vi "Display.vi"(0 "STEP in":refnum<class "STEP.lvclass">, 2 "Alarms triggered?":T3, 3 "STEP State":T4, 4 "Current Sequence":T1, 5 "error in (no error)":errorcluster, 9 "SEQ STEP Display":refnum<notifier>) -> (14 "STEP out":refnum<class "STEP.lvclass">, 19 "error out":errorcluster)   [LabVIEW 2014, in "SeqLoop.lvlib" / "STEP Classes.lvlib" / "STEP.lvclass"]
doc: "Gestiona el envío de Datos al Display."
uses:
  STEP.lvclass
  TypeDefs/STEP State.ctl
  TypeDefs/STEP Display.ctl
  Mimico Display/TypeDefs/Mimic Data.ctl
  Mimico Display/TypeDefs/BG Image.ctl
  Mimico Display/TypeDefs/mObject.ctl
  TypeDefs/Sequence.ctl
  TypeDefs/LogicParsedExpression.ctl
  STEP.lvclass/STEP.ctl
  Mimico Display/Mimico Display.lvlib
  SeqLoop.lvlib
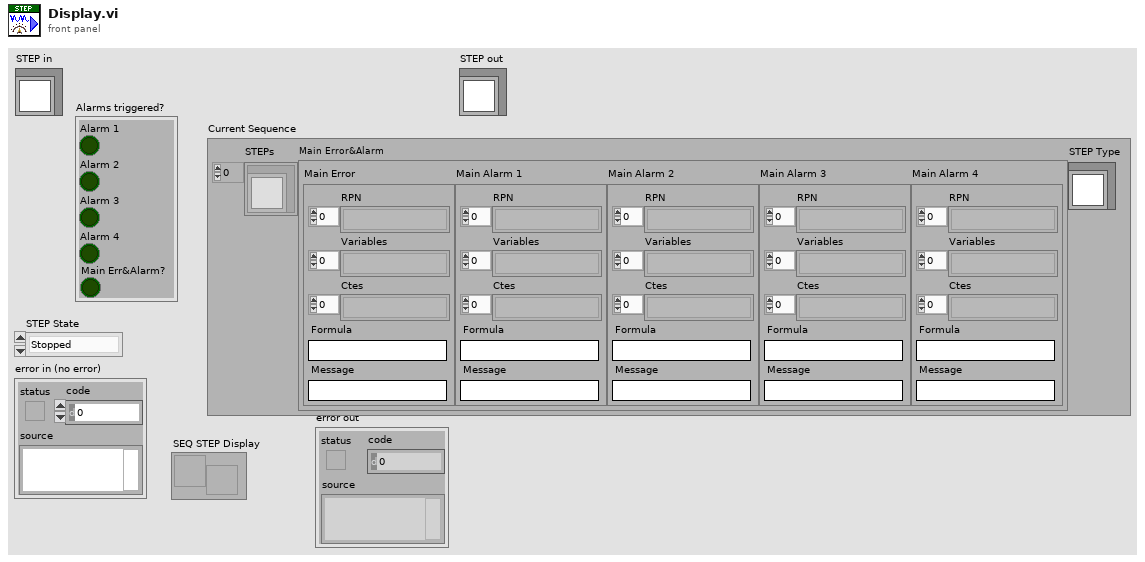
[diagram p1: front panel]
types:
  T1 = typedef "SeqLoop.lvlib/Sequence.ctl" = cluster{"STEPs":refnum<class "STEP.lvclass">[], "Main Error&Alarm":cluster{"Main Error":T2, "Main Alarm 1":T2, "Main Alarm 2":T2, "Main Alarm 3":T2, "Main Alarm 4":T2}, "STEP Type":refnum<class "STEP.lvclass">}
  T2 = typedef "SeqLoop.lvlib/LogicParsedExpression.ctl" = cluster{"RPN ":string[], "Variables":string[], "Ctes":string[], "Formula":string, "Message":string}
  T3 = cluster{"Alarm 1":bool, "Alarm 2":bool, "Alarm 3":bool, "Alarm 4":bool, "Main Err&Alarm?":bool}
  T4 = typedef "SeqLoop.lvlib/STEP State.ctl" = enum16{"Stopped", "First Call", "Idle...", "Advance OK", "Alarm", "Output Security", "Error"}
  T5 = typedef "STEP Display.ctl" = cluster{"Mimic Data":T6, "Operator Mssg":string, "Error":cluster{"true?":bool, "Message":string}, "Alarm 1":cluster{"true?":bool, "Message":string}, "Alarm 2":cluster{"true?":bool, "Message":string}, "Alarm 3":cluster{"true?":bool, "Message":string}, "Alarm 4":cluster{"true?":bool, "Message":string}}
  T6 = typedef "SeqLoop.lvlib/Mimico Display.lvlib/Mimic Data.ctl" = cluster{"BG Image":T7, "Mimic mObjects":T8[]}
  T7 = typedef "SeqLoop.lvlib/Mimico Display.lvlib/BG Image.ctl" = cluster{"Path":path, "point":cluster{"x":i16, "y":i16}}
  T8 = typedef "SeqLoop.lvlib/Mimico Display.lvlib/mObject.ctl" = cluster{"point":cluster{"x":i16, "y":i16}, "Precision (Digits)":i32, "Visible?":bool, "Ref":string, "Comment":string}
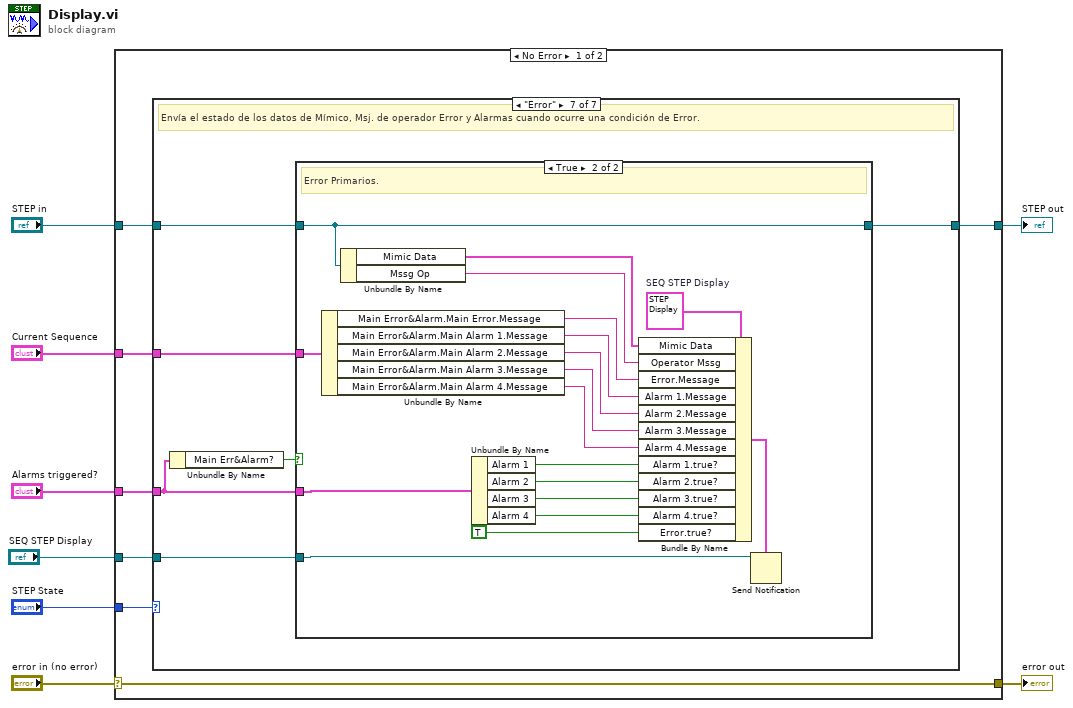
[diagram p0: block diagram]
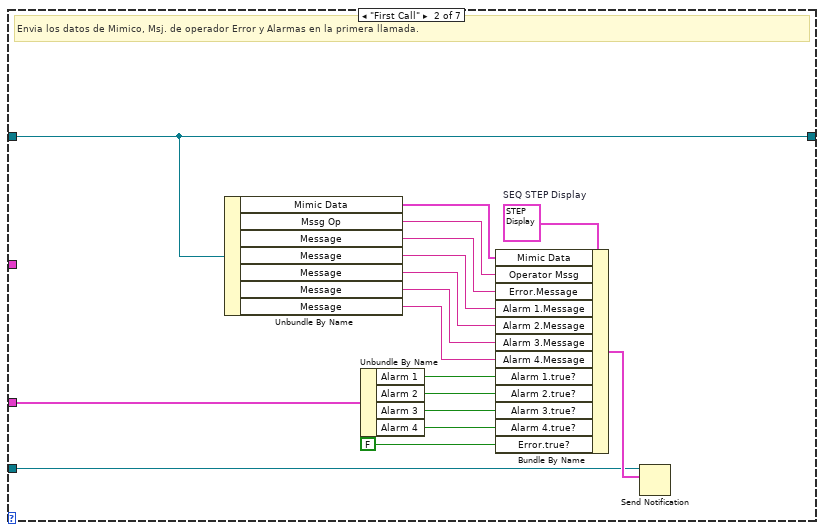
[diagram p3: hidden frame]
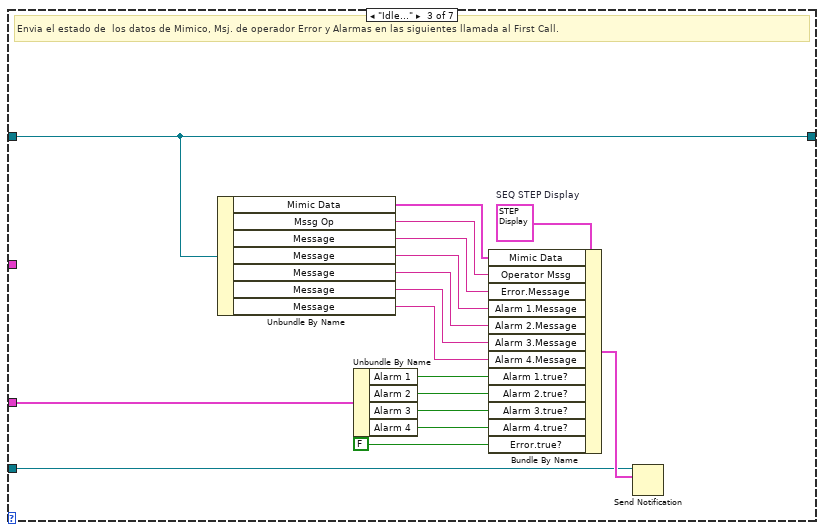
[diagram p4: hidden frame]
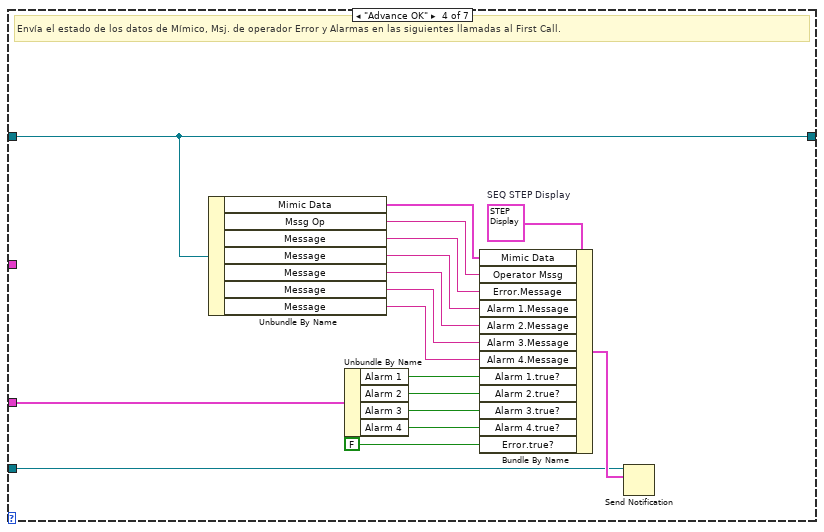
[diagram p5: hidden frame]
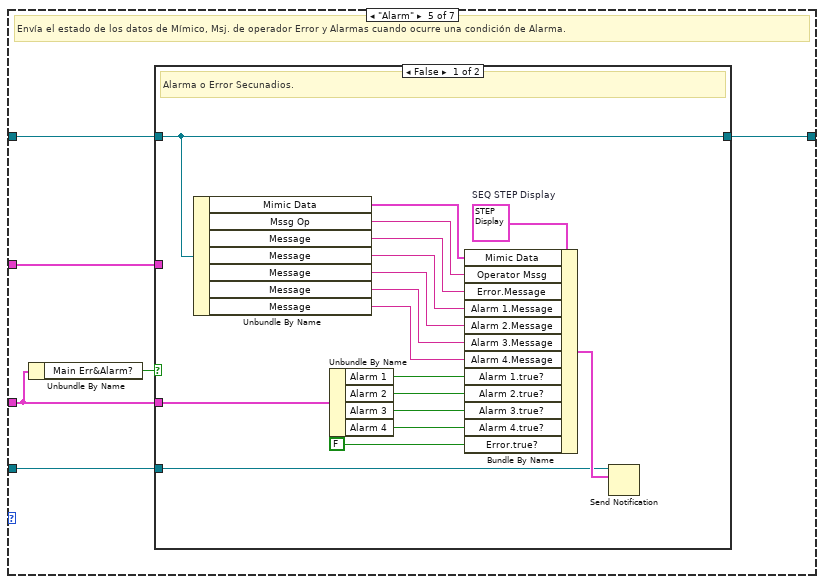
[diagram p6: hidden frame]
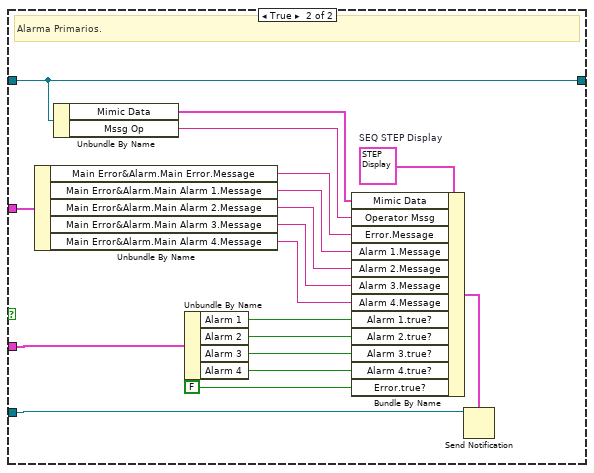
[diagram p7: hidden frame]
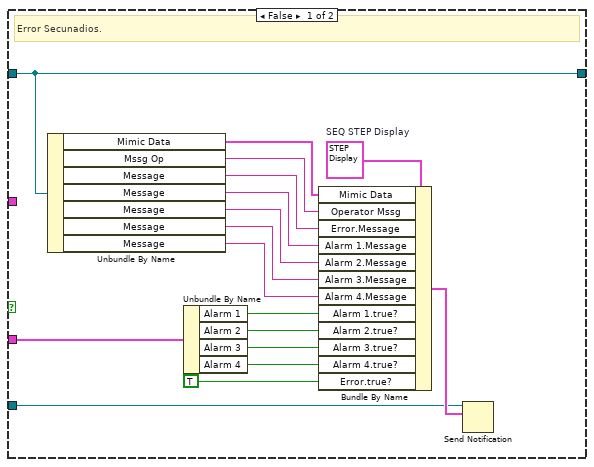
[diagram p9: hidden frame]
diagram:
  n1 = case shown="No Error" "error in (no error)" {
    selector: "error in (no error)" -> [w15 w152]
    tunnel: [w15 w152] -> w7
    tunnel: [w13 w151] -> w5
    tunnel: "STEP in" -> [w14 w151]
    tunnel: "STEP State" -> [w12 _]
    tunnel: "Alarms triggered?" -> [w11 _]
    tunnel: "SEQ STEP Display" -> [w10 _]
    tunnel: "Current Sequence" -> [w9 _]
    frame No Error {
      n2 = case shown="\"Error\"" w12 {
        tunnel: w14 -> [w16 w17 w34 w52 w72 w109 w115]
        tunnel: [w16 w17 w34 w52 w68 w109 w110] -> w13
        tunnel: w11 -> [_ w18 w36 w53 w70 _ w113]
        tunnel: w10 -> [_ w19 w35 w51 w69 _ w114]
        tunnel: w9 -> [_ _ _ _ w71 _ w111]
        frame "Stopped", Default {
        }
        frame "First Call" {
          w33 = T5 {"Mimic Data"={"BG Image"={"Path"=path "", "point"={"x"=0, "y"=0}}, "Mimic mObjects"=[]}, "Operator Mssg"="", "Error"={"true?"=FALSE, "Message"=""}, "Alarm 1"={"true?"=FALSE, "Message"=""}, "Alarm 2"={"true?"=FALSE, "Message"=""}, "Alarm 3"={"true?"=FALSE, "Message"=""}, "Alarm 4"={"true?"=FALSE, "Message"=""}}  # SEQ STEP Display
          # "Envia los datos de Mimico, Msj. de operador Error y Alarmas en la primera llamada."
          n3 = Unbundle By Name(w17) -> ("Mimic Data"=w32:T6, "Mssg Op"=w31:string, "Message"=w30:string, "Message"=w29:string, "Message"=w28:string, "Message"=w27:string, "Message"=w26:string)
          n4 = Unbundle By Name(w18) -> ("Alarm 1"=w25:bool, "Alarm 2"=w24:bool, "Alarm 3"=w23:bool, "Alarm 4"=w22:bool)
          n5 = Bundle By Name(cluster=w33, "Mimic Data"=w32, "Operator Mssg"=w31, "Error.Message"=w30, "Alarm 1.Message"=w29, "Alarm 2.Message"=w28, "Alarm 3.Message"=w27, "Alarm 4.Message"=w26, "Alarm 1.true?"=w25, "Alarm 2.true?"=w24, "Alarm 3.true?"=w23, "Alarm 4.true?"=w22, "Error.true?"=FALSE) -> (w21:T5)
          n6 = Send Notification(notification=w21, notifier=w19) -> ()  [unwired: 1 in, 2 out]
        }
        frame "Idle..." {
          w37 = T5 {"Mimic Data"={"BG Image"={"Path"=path "", "point"={"x"=0, "y"=0}}, "Mimic mObjects"=[]}, "Operator Mssg"="", "Error"={"true?"=FALSE, "Message"=""}, "Alarm 1"={"true?"=FALSE, "Message"=""}, "Alarm 2"={"true?"=FALSE, "Message"=""}, "Alarm 3"={"true?"=FALSE, "Message"=""}, "Alarm 4"={"true?"=FALSE, "Message"=""}}  # SEQ STEP Display
          # "Envia el estado de  los datos de Mimico, Msj. de operador Error y Alarmas en las siguientes llamada al First Call."
          n7 = Unbundle By Name(w34) -> ("Mimic Data"=w38:T6, "Mssg Op"=w39:string, "Message"=w40:string, "Message"=w41:string, "Message"=w42:string, "Message"=w43:string, "Message"=w44:string)
          n8 = Unbundle By Name(w36) -> ("Alarm 1"=w45:bool, "Alarm 2"=w46:bool, "Alarm 3"=w47:bool, "Alarm 4"=w48:bool)
          n9 = Bundle By Name(cluster=w37, "Mimic Data"=w38, "Operator Mssg"=w39, "Error.Message"=w40, "Alarm 1.Message"=w41, "Alarm 2.Message"=w42, "Alarm 3.Message"=w43, "Alarm 4.Message"=w44, "Alarm 1.true?"=w45, "Alarm 2.true?"=w46, "Alarm 3.true?"=w47, "Alarm 4.true?"=w48, "Error.true?"=FALSE) -> (w49:T5)
          n10 = Send Notification(notification=w49, notifier=w35) -> ()  [unwired: 1 in, 2 out]
        }
        frame "Advance OK" {
          w67 = T5 {"Mimic Data"={"BG Image"={"Path"=path "", "point"={"x"=0, "y"=0}}, "Mimic mObjects"=[]}, "Operator Mssg"="", "Error"={"true?"=FALSE, "Message"=""}, "Alarm 1"={"true?"=FALSE, "Message"=""}, "Alarm 2"={"true?"=FALSE, "Message"=""}, "Alarm 3"={"true?"=FALSE, "Message"=""}, "Alarm 4"={"true?"=FALSE, "Message"=""}}  # SEQ STEP Display
          # "Envía el estado de los datos de Mímico, Msj. de operador Error y Alarmas en las siguientes llamadas al First Call."
          n11 = Unbundle By Name(w52) -> ("Mimic Data"=w66:T6, "Mssg Op"=w65:string, "Message"=w64:string, "Message"=w63:string, "Message"=w62:string, "Message"=w61:string, "Message"=w60:string)
          n12 = Unbundle By Name(w53) -> ("Alarm 1"=w59:bool, "Alarm 2"=w58:bool, "Alarm 3"=w57:bool, "Alarm 4"=w56:bool)
          n13 = Bundle By Name(cluster=w67, "Mimic Data"=w66, "Operator Mssg"=w65, "Error.Message"=w64, "Alarm 1.Message"=w63, "Alarm 2.Message"=w62, "Alarm 3.Message"=w61, "Alarm 4.Message"=w60, "Alarm 1.true?"=w59, "Alarm 2.true?"=w58, "Alarm 3.true?"=w57, "Alarm 4.true?"=w56, "Error.true?"=FALSE) -> (w55:T5)
          n14 = Send Notification(notification=w55, notifier=w51) -> ()  [unwired: 1 in, 2 out]
        }
        frame "Alarm" {
          # "Envía el estado de los datos de Mímico, Msj. de operador Error y Alarmas cuando ocurre una condición de Alarma."
          n15 = Unbundle By Name(w70) -> ("Main Err&Alarm?"=w73:bool)
          n16 = case shown="False" w73 {
            tunnel: w72 -> [w74 w91]
            tunnel: w69 -> [w77 w94]
            tunnel: w70 -> [w75 w95]
            tunnel: w71 -> [_ w96]
            tunnel: [w74 w91] -> w68
            frame False {
              w90 = T5 {"Mimic Data"={"BG Image"={"Path"=path "", "point"={"x"=0, "y"=0}}, "Mimic mObjects"=[]}, "Operator Mssg"="", "Error"={"true?"=FALSE, "Message"=""}, "Alarm 1"={"true?"=FALSE, "Message"=""}, "Alarm 2"={"true?"=FALSE, "Message"=""}, "Alarm 3"={"true?"=FALSE, "Message"=""}, "Alarm 4"={"true?"=FALSE, "Message"=""}}  # SEQ STEP Display
              # "Alarma o Error Secunadios."
              n17 = Unbundle By Name(w74) -> ("Mimic Data"=w89:T6, "Mssg Op"=w88:string, "Message"=w87:string, "Message"=w86:string, "Message"=w85:string, "Message"=w84:string, "Message"=w83:string)
              n18 = Unbundle By Name(w75) -> ("Alarm 1"=w82:bool, "Alarm 2"=w81:bool, "Alarm 3"=w80:bool, "Alarm 4"=w79:bool)
              n19 = Bundle By Name(cluster=w90, "Mimic Data"=w89, "Operator Mssg"=w88, "Error.Message"=w87, "Alarm 1.Message"=w86, "Alarm 2.Message"=w85, "Alarm 3.Message"=w84, "Alarm 4.Message"=w83, "Alarm 1.true?"=w82, "Alarm 2.true?"=w81, "Alarm 3.true?"=w80, "Alarm 4.true?"=w79, "Error.true?"=FALSE) -> (w78:T5)
              n20 = Send Notification(notification=w78, notifier=w77) -> ()  [unwired: 1 in, 2 out]
            }
            frame True {
              w108 = T5 {"Mimic Data"={"BG Image"={"Path"=path "", "point"={"x"=0, "y"=0}}, "Mimic mObjects"=[]}, "Operator Mssg"="", "Error"={"true?"=FALSE, "Message"=""}, "Alarm 1"={"true?"=FALSE, "Message"=""}, "Alarm 2"={"true?"=FALSE, "Message"=""}, "Alarm 3"={"true?"=FALSE, "Message"=""}, "Alarm 4"={"true?"=FALSE, "Message"=""}}  # SEQ STEP Display
              # "Alarma Primarios."
              n21 = Unbundle By Name(w96) -> ("Main Error&Alarm.Main Error.Message"=w107:string, "Main Error&Alarm.Main Alarm 1.Message"=w106:string, "Main Error&Alarm.Main Alarm 2.Message"=w105:string, "Main Error&Alarm.Main Alarm 3.Message"=w104:string, "Main Error&Alarm.Main Alarm 4.Message"=w103:string)
              n22 = Unbundle By Name(w91) -> ("Mimic Data"=w93:T6, "Mssg Op"=w92:string)
              n23 = Unbundle By Name(w95) -> ("Alarm 1"=w102:bool, "Alarm 2"=w101:bool, "Alarm 3"=w100:bool, "Alarm 4"=w99:bool)
              n24 = Bundle By Name(cluster=w108, "Mimic Data"=w93, "Operator Mssg"=w92, "Error.Message"=w107, "Alarm 1.Message"=w106, "Alarm 2.Message"=w105, "Alarm 3.Message"=w104, "Alarm 4.Message"=w103, "Alarm 1.true?"=w102, "Alarm 2.true?"=w101, "Alarm 3.true?"=w100, "Alarm 4.true?"=w99, "Error.true?"=FALSE) -> (w98:T5)
              n25 = Send Notification(notification=w98, notifier=w94) -> ()  [unwired: 1 in, 2 out]
            }
          }
        }
        frame "Output Security" {
        }
        frame "Error" {
          # "Envía el estado de los datos de Mímico, Msj. de operador Error y Alarmas cuando ocurre una condición de Error."
          n26 = Unbundle By Name(w113) -> ("Main Err&Alarm?"=w112:bool)
          n27 = case shown="True" w112 {
            tunnel: w115 -> [w116 w133]
            tunnel: w114 -> [w119 w136]
            tunnel: w113 -> [w117 w137]
            tunnel: w111 -> [_ w138]
            tunnel: [w116 w133] -> w110
            frame False {
              w132 = T5 {"Mimic Data"={"BG Image"={"Path"=path "", "point"={"x"=0, "y"=0}}, "Mimic mObjects"=[]}, "Operator Mssg"="", "Error"={"true?"=FALSE, "Message"=""}, "Alarm 1"={"true?"=FALSE, "Message"=""}, "Alarm 2"={"true?"=FALSE, "Message"=""}, "Alarm 3"={"true?"=FALSE, "Message"=""}, "Alarm 4"={"true?"=FALSE, "Message"=""}}  # SEQ STEP Display
              # "Error Secunadios."
              n28 = Unbundle By Name(w116) -> ("Mimic Data"=w131:T6, "Mssg Op"=w130:string, "Message"=w129:string, "Message"=w128:string, "Message"=w127:string, "Message"=w126:string, "Message"=w125:string)
              n29 = Unbundle By Name(w117) -> ("Alarm 1"=w124:bool, "Alarm 2"=w123:bool, "Alarm 3"=w122:bool, "Alarm 4"=w121:bool)
              n30 = Bundle By Name(cluster=w132, "Mimic Data"=w131, "Operator Mssg"=w130, "Error.Message"=w129, "Alarm 1.Message"=w128, "Alarm 2.Message"=w127, "Alarm 3.Message"=w126, "Alarm 4.Message"=w125, "Alarm 1.true?"=w124, "Alarm 2.true?"=w123, "Alarm 3.true?"=w122, "Alarm 4.true?"=w121, "Error.true?"=TRUE) -> (w120:T5)
              n31 = Send Notification(notification=w120, notifier=w119) -> ()  [unwired: 1 in, 2 out]
            }
            frame True {
              w150 = T5 {"Mimic Data"={"BG Image"={"Path"=path "", "point"={"x"=0, "y"=0}}, "Mimic mObjects"=[]}, "Operator Mssg"="", "Error"={"true?"=FALSE, "Message"=""}, "Alarm 1"={"true?"=FALSE, "Message"=""}, "Alarm 2"={"true?"=FALSE, "Message"=""}, "Alarm 3"={"true?"=FALSE, "Message"=""}, "Alarm 4"={"true?"=FALSE, "Message"=""}}  # SEQ STEP Display
              # "Error Primarios."
              n32 = Unbundle By Name(w138) -> ("Main Error&Alarm.Main Error.Message"=w149:string, "Main Error&Alarm.Main Alarm 1.Message"=w148:string, "Main Error&Alarm.Main Alarm 2.Message"=w147:string, "Main Error&Alarm.Main Alarm 3.Message"=w146:string, "Main Error&Alarm.Main Alarm 4.Message"=w145:string)
              n33 = Unbundle By Name(w133) -> ("Mimic Data"=w135:T6, "Mssg Op"=w134:string)
              n34 = Unbundle By Name(w137) -> ("Alarm 1"=w144:bool, "Alarm 2"=w143:bool, "Alarm 3"=w142:bool, "Alarm 4"=w141:bool)
              n35 = Bundle By Name(cluster=w150, "Mimic Data"=w135, "Operator Mssg"=w134, "Error.Message"=w149, "Alarm 1.Message"=w148, "Alarm 2.Message"=w147, "Alarm 3.Message"=w146, "Alarm 4.Message"=w145, "Alarm 1.true?"=w144, "Alarm 2.true?"=w143, "Alarm 3.true?"=w142, "Alarm 4.true?"=w141, "Error.true?"=TRUE) -> (w140:T5)
              n36 = Send Notification(notification=w140, notifier=w136) -> ()  [unwired: 1 in, 2 out]
            }
          }
        }
      }
    }
    frame Error {
    }
  }
  "error out" <- w7
  "STEP out" <- w5
